vi "WSVCAP SHL FPGA LL I2C Read Data.vi"(11 "error in (no error)":errorcluster, 12 "UUT Set (0-1)":u8, 13 "Socket Mask":u64 format="%012x") -> (4 "Long Word Out (1-Bit for Each Channel)":u64, 15 "error out":errorcluster)   [LabVIEW 2012]
uses:
  WSVCAP SHL FPGA LL I2C Debug Global.vi
  <vilib>/eio/EIONode/EIONode.xnode
  <vilib>/rvi/eio/common/nirviEmuTemplateMethod_errors.vi
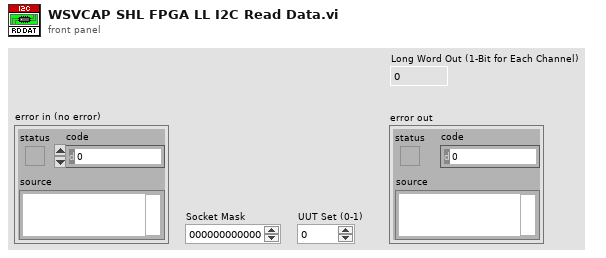
[diagram p1: front panel]
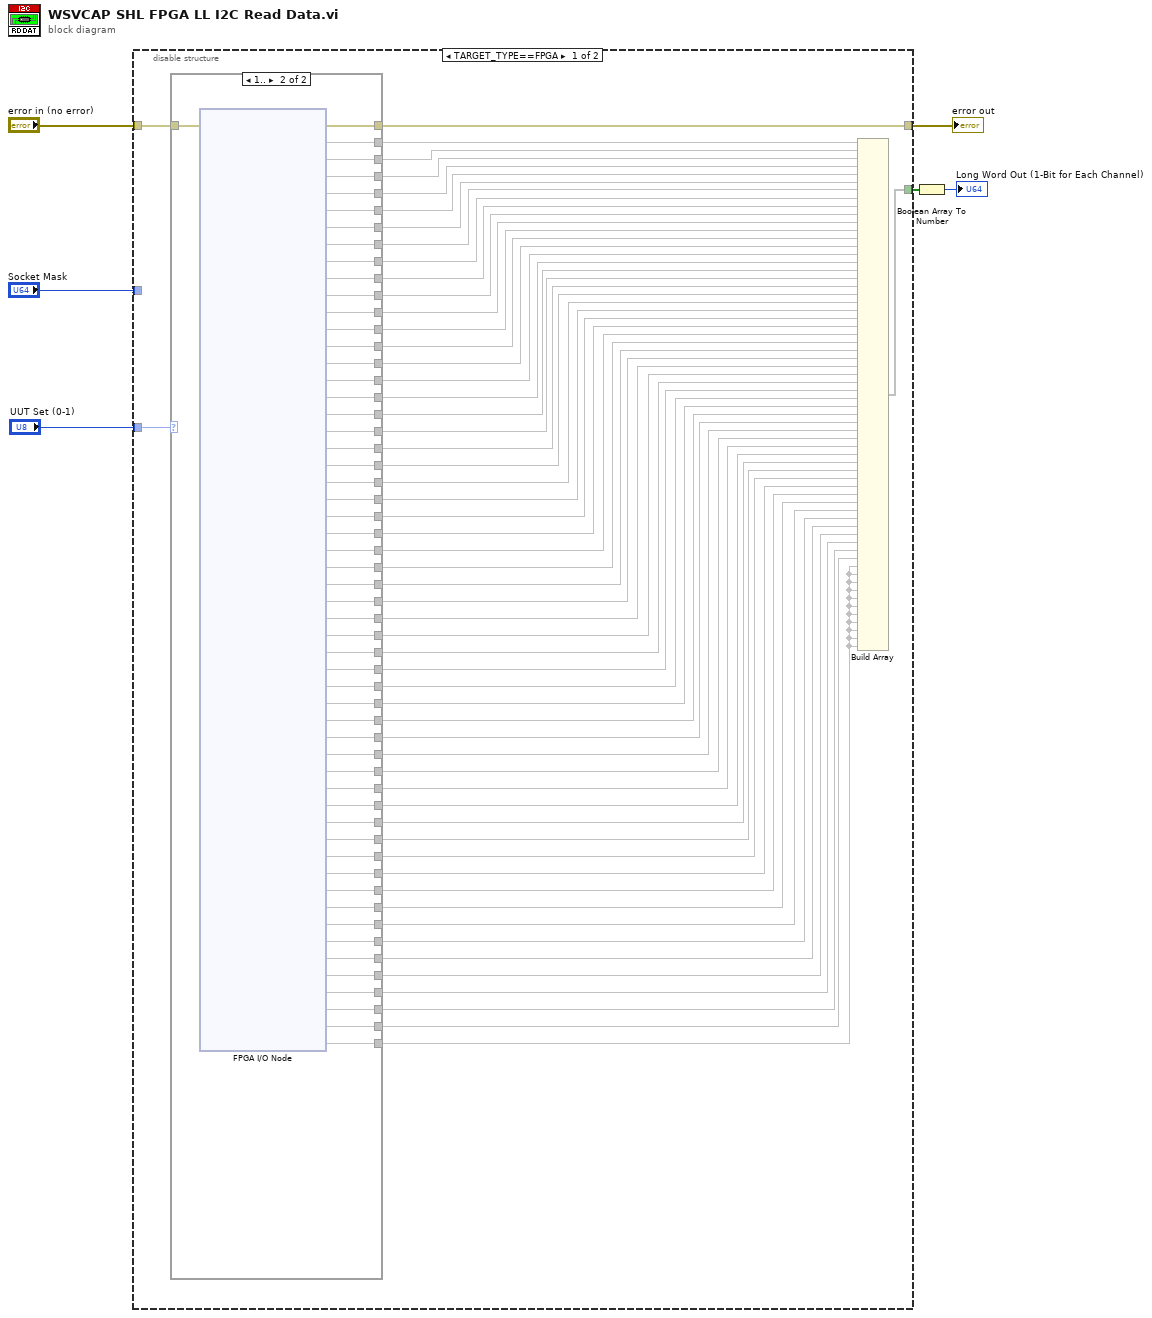
[diagram p0: block diagram]
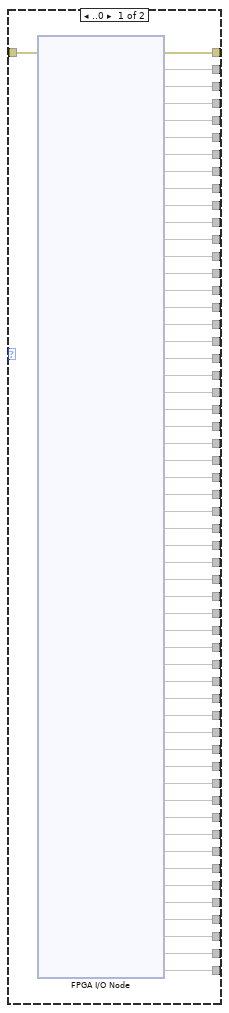
[diagram p2: hidden frame]
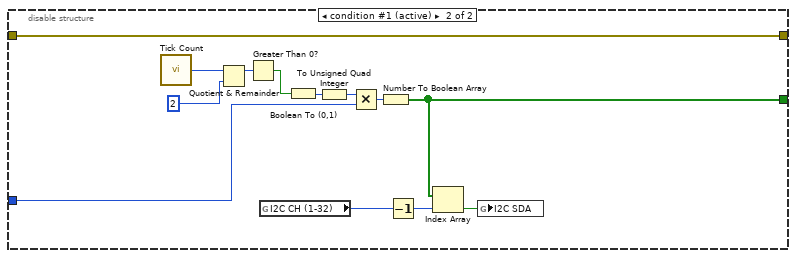
[diagram p3: hidden frame]
diagram:
  n1 = disable-structure shown="TARGET_TYPE==FPGA" {
    disable-tunnel: [w64 w186] -> w6
    disable-tunnel: "error in (no error)" -> [w63 w186]
    disable-tunnel: "Socket Mask" -> [_ w183]
    disable-tunnel: [w29 w177] -> w2
    disable-tunnel: "UUT Set (0-1)" -> [w26 _]
    frame condition #0 {
      n2 = case shown="1.." w26 {
        tunnel: [w120 w176] -> w64
        tunnel: w63 -> [w119 w175]
        tunnel: [w118 w174] -> w62
        tunnel: [w117 w173] -> w61
        tunnel: [w116 w172] -> w60
        tunnel: [w115 w171] -> w59
        tunnel: [w114 w170] -> w58
        tunnel: [w113 w169] -> w57
        tunnel: [w112 w168] -> w56
        tunnel: [w111 w167] -> w55
        tunnel: [w110 w166] -> w54
        tunnel: [w109 w165] -> w53
        tunnel: [w108 w164] -> w52
        tunnel: [w107 w163] -> w51
        tunnel: [w106 w162] -> w50
        tunnel: [w105 w161] -> w49
        tunnel: [w104 w160] -> w48
        tunnel: [w103 w159] -> w47
        tunnel: [w102 w158] -> w46
        tunnel: [w101 w157] -> w45
        tunnel: [w100 w156] -> w44
        tunnel: [w99 w155] -> w43
        tunnel: [w98 w154] -> w42
        tunnel: [w97 w153] -> w41
        tunnel: [w96 w152] -> w40
        tunnel: [w95 w151] -> w39
        tunnel: [w94 w150] -> w38
        tunnel: [w93 w149] -> w37
        tunnel: [w92 w148] -> w36
        tunnel: [w91 w147] -> w35
        tunnel: [w90 w146] -> w34
        tunnel: [w89 w145] -> w33
        tunnel: [w88 w144] -> w32
        tunnel: [w87 w143] -> w31
        tunnel: [w86 w142] -> w30
        tunnel: [w85 w141] -> w28
        tunnel: [w84 w140] -> w27
        tunnel: [w83 w139] -> w25
        tunnel: [w82 w138] -> w24
        tunnel: [w81 w137] -> w23
        tunnel: [w80 w136] -> w22
        tunnel: [w79 w135] -> w21
        tunnel: [w78 w134] -> w20
        tunnel: [w77 w133] -> w19
        tunnel: [w76 w132] -> w18
        tunnel: [w75 w131] -> w17
        tunnel: [w74 w130] -> w16
        tunnel: [w73 w129] -> w15
        tunnel: [w72 w128] -> w14
        tunnel: [w71 w127] -> w13
        tunnel: [w70 w126] -> w12
        tunnel: [w69 w125] -> w11
        tunnel: [w68 w124] -> w10
        tunnel: [w67 w123] -> w9
        tunnel: [w66 w122] -> w8
        tunnel: [w65 w121] -> w7
        frame ..0 {
          n3 = xnode "FPGA I/O Node"("error in"=w119) -> ("error out"=w120:errorcluster, "I2C_SDA_C1_S1"=w118, "I2C_SDA_C1_S2"=w117, "I2C_SDA_C1_S3"=w116, "I2C_SDA_C1_S4"=w115, "I2C_SDA_C1_S5"=w114, "I2C_SDA_C1_S6"=w113, "I2C_SDA_C1_S7"=w112, "I2C_SDA_C1_S8"=w111, "I2C_SDA_C1_S9"=w110, "I2C_SDA_C1_S10"=w109, "I2C_SDA_C1_S11"=w108, "I2C_SDA_C1_S12"=w107, "I2C_SDA_C1_S13"=w106, "I2C_SDA_C1_S14"=w105, "I2C_SDA_C1_S15"=w104, "I2C_SDA_C1_S16"=w85, "I2C_SDA_C1_S17"=w84, "I2C_SDA_C1_S18"=w103, "I2C_SDA_C2_S1"=w102, "I2C_SDA_C2_S2"=w101, "I2C_SDA_C2_S3"=w100, "I2C_SDA_C2_S4"=w99, "I2C_SDA_C2_S5"=w98, "I2C_SDA_C2_S6"=w97, "I2C_SDA_C2_S7"=w96, "I2C_SDA_C2_S8"=w95, "I2C_SDA_C2_S9"=w94, "I2C_SDA_C2_S10"=w93, "I2C_SDA_C2_S11"=w92, "I2C_SDA_C2_S12"=w91, "I2C_SDA_C2_S13"=w90, "I2C_SDA_C2_S14"=w89, "I2C_SDA_C2_S15"=w88, "I2C_SDA_C2_S16"=w87, "I2C_SDA_C2_S17"=w86, "I2C_SDA_C2_S18"=w83, "I2C_SDA_C3_S1"=w82, "I2C_SDA_C3_S2"=w81, "I2C_SDA_C3_S3"=w80, "I2C_SDA_C3_S4"=w79, "I2C_SDA_C3_S5"=w78, "I2C_SDA_C3_S6"=w77, "I2C_SDA_C3_S7"=w76, "I2C_SDA_C3_S8"=w75, "I2C_SDA_C3_S9"=w74, "I2C_SDA_C3_S10"=w73, "I2C_SDA_C3_S11"=w72, "I2C_SDA_C3_S12"=w71, "I2C_SDA_C3_S13"=w70, "I2C_SDA_C3_S14"=w69, "I2C_SDA_C3_S15"=w68, "I2C_SDA_C3_S16"=w67, "I2C_SDA_C3_S17"=w66, "I2C_SDA_C3_S18"=w65)  [unwired: 54 in, 54 out]
        }
        frame 1.. {
          n4 = xnode "FPGA I/O Node"("error in"=w175) -> ("error out"=w176:errorcluster, "I2C_SDA_C1_S19"=w174, "I2C_SDA_C1_S20"=w173, "I2C_SDA_C1_S21"=w172, "I2C_SDA_C1_S22"=w171, "I2C_SDA_C1_S23"=w170, "I2C_SDA_C1_S24"=w169, "I2C_SDA_C1_S25"=w168, "I2C_SDA_C1_S26"=w167, "I2C_SDA_C1_S27"=w166, "I2C_SDA_C1_S28"=w165, "I2C_SDA_C1_S29"=w164, "I2C_SDA_C1_S30"=w163, "I2C_SDA_C1_S31"=w162, "I2C_SDA_C1_S32"=w161, "I2C_SDA_C1_S33"=w160, "I2C_SDA_C1_S34"=w141, "I2C_SDA_C1_S35"=w140, "I2C_SDA_C1_S36"=w159, "I2C_SDA_C2_S19"=w158, "I2C_SDA_C2_S20"=w157, "I2C_SDA_C2_S21"=w156, "I2C_SDA_C2_S22"=w155, "I2C_SDA_C2_S23"=w154, "I2C_SDA_C2_S24"=w153, "I2C_SDA_C2_S25"=w152, "I2C_SDA_C2_S26"=w151, "I2C_SDA_C2_S27"=w150, "I2C_SDA_C2_S28"=w149, "I2C_SDA_C2_S29"=w148, "I2C_SDA_C2_S30"=w147, "I2C_SDA_C2_S31"=w146, "I2C_SDA_C2_S32"=w145, "I2C_SDA_C2_S33"=w144, "I2C_SDA_C2_S34"=w143, "I2C_SDA_C2_S35"=w142, "I2C_SDA_C2_S36"=w139, "I2C_SDA_C3_S19"=w138, "I2C_SDA_C3_S20"=w137, "I2C_SDA_C3_S21"=w136, "I2C_SDA_C3_S22"=w135, "I2C_SDA_C3_S23"=w134, "I2C_SDA_C3_S24"=w133, "I2C_SDA_C3-S25"=w132, "I2C_SDA_C3_S26"=w131, "I2C_SDA_C3_S27"=w130, "I2C_SDA_C3_S28"=w129, "I2C_SDA_C3_S29"=w128, "I2C_SDA_C3_S30"=w127, "I2C_SDA_C3_S31"=w126, "I2C_SDA_C3_S32"=w125, "I2C_SDA_C3_S33"=w124, "I2C_SDA_C3_S34"=w123, "I2C_SDA_C3_S35"=w122, "I2C_SDA_C3_S36"=w121)  [unwired: 54 in, 54 out]
        }
      }
      n5 = Build Array(w62, w61, w60, w59, w58, w57, w56, w55, w54, w53, w52, w51, w50, w49, w48, w28, w27, w47, w46, w45, w44, w43, w42, w41, w40, w39, w38, w37, w36, w35, w34, w33, w32, w31, w30, w25, w24, w23, w22, w21, w20, w19, w18, w17, w16, w15, w14, w13, w12, w11, w10, w9, w8, w7, w7, w7, w7, w7, w7, w7, w7, w7, w7, w7) -> (w29:void[])
    }
    frame condition #1 (active) {
      n6 = call "Tick Count"() -> ("Tick Count(Ticks)"=w189:u32)
      n7 = Quotient & Remainder(x=w189, y=u32 2) -> (x-y*floor(x/y)=w188:u32)  [unwired: 1 out]
      n8 = Greater Than 0?(x=w188) -> (x > 0?=w185:bool)
      n9 = global read "WSVCAP SHL FPGA LL I2C Debug Global.vi" "I2C CH (1-32)"() -> (w182:i32)
      n10 = Boolean To (0,1)(Boolean=w185) -> (0, 1=w184:i16)
      n11 = To Unsigned Quad Integer(1:w184) -> (0:w181:u64)
      n12 = Multiply(x=w181, y=w183) -> (x*y=w180:u64)
      n13 = Number To Boolean Array(number=w180) -> (Boolean array=w177:bool[])
      n14 = Decrement(x=w182) -> (x-1=w178:i32)
      n15 = Index Array(array=w177, index=w178) -> (element=w179:bool)
      n16 = global write "WSVCAP SHL FPGA LL I2C Debug Global.vi" "I2C SDA"(w179) -> ()
    }
  }
  "error out" <- w6
  n17 = Boolean Array To Number(Boolean array=w2) -> (number=→"Long Word Out (1-Bit for Each Channel)":u64)
